vi "DOS cmd.vi"(8 "错误输入（无错误）":errorcluster) -> (0 "error out":errorcluster caption="错误输出")   [LabVIEW 2016, in "数据传输系统.lvlib" / "update.lvlib"]
uses:
  update.lvlib
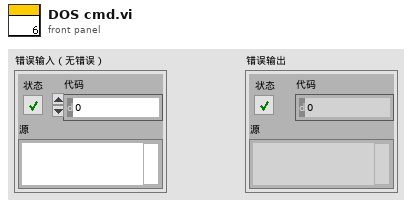
[diagram p1: front panel]
types:
  T1 = enum16{"open", "replace", "create", "open or create", "replace or create", "replace or create with confirmation"}
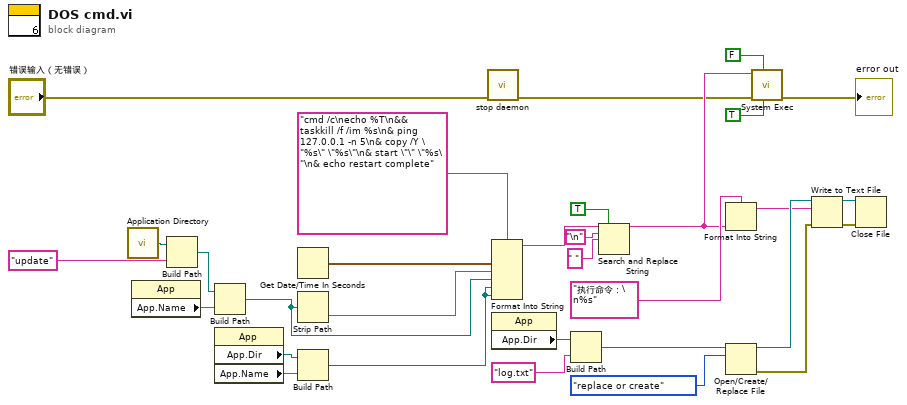
[diagram p0: block diagram]
diagram:
  n1 = call <vilib>:"Application Directory.vi"() -> ("Application Directory"=w17:path)
  n2 = property class="App"() -> ("App.Name"=w14:string)  [unwired: 2 in, 2 out]
  n3 = Build Path(base path=w17, name or relative path="update" ("名称或相对路径")) -> (appended path=w15:path)
  n4 = Build Path(base path=w15, name or relative path=w14) -> (appended path=w11:path)
  n5 = property class="App"() -> ("App.Dir"=w13:path, "App.Name"=w12:string)  [unwired: 2 in, 2 out]
  n6 = Get Date/Time In Seconds() -> (seconds since 1Jan1904=w18:timestamp)
  n7 = Strip Path(path=w11) -> (name=w19:string)  [unwired: 1 out]
  n8 = Build Path(base path=w13, name or relative path=w12) -> (appended path=w10:path)
  n9 = call "stop daemon.vi"("error in (no error)"="错误输入（无错误）") -> ("error out"=w1:errorcluster)  [unwired: 10 in]
  n10 = Format Into String(format string="cmd /c\necho %T\n&& taskkill /f /im %s\n& ping 127.0.0.1 -n 5\n& copy /Y \"%s\" \"%s\"\n& start \"\" \"%s\"\n& echo restart complete" ("文本"), w18, w19, w11, w10, w10) -> (resulting string=w7:string)  [unwired: 2 in, 1 out]
  n11 = property class="App"() -> ("App.Dir"=w26:path)  [unwired: 2 in, 2 out]
  n12 = Build Path(base path=w26, name or relative path="log.txt" ("名称或相对路径")) -> (appended path=w24:path)
  n13 = Search and Replace String(replace all?=TRUE ("替换全部？(F)"), input string=w7, search string="\n", replace string=" " ("替换字符串(\"\")")) -> (result string=w4:string)  [unwired: 4 in, 3 out]
  n14 = Format Into String(format string="执行命令：\n%s" ("格式字符串"), w4) -> (resulting string=w21:string)  [unwired: 2 in, 1 out]
  n15 = Open/Create/Replace File(file path (use dialog)=w24, operation (0:open)=T1."replace or create" ("操作(0:open)")) -> (refnum out=w27:refnum<file>, error out=w30:errorcluster)  [unwired: 4 in, 1 out]
  n16 = call <vilib>:"System Exec.vi"("run minimized? (F)"=TRUE, "wait until completion? (T)"=FALSE, "error in (no error)"=w1, "command line"=w4) -> ("error out"=→"error out":errorcluster)  [unwired: 4 in, 3 out]
  n17 = Write to Text File(file (use dialog)=w27, text=w21, error in=w30) -> (refnum out=w28:refnum<file>, error out=w29:errorcluster)  [unwired: 1 in, 1 out]
  n18 = Close File(refnum=w28, error in=w29) -> ()  [unwired: 2 out]
